vi "Parse Signal List.vi"(8 "error in (no error)":errorcluster, 11 "SwitchMatrix in":refnum<class "SwitchMatrix.lvclass">) -> (0 "error out":errorcluster, 3 "SwitchMatrix out":refnum<class "SwitchMatrix.lvclass">)   [LabVIEW 2019, in "SwitchMatrix.lvlib" / "SwitchMatrix.lvclass"]
uses:
  Library/SwitchMatrix.lvclass
  C:/Users/Public/Documents/Development/builds/Tools/Config.lvlibp/Config.lvclass
  Library/SwitchMatrix.lvclass/SwitchMatrix.ctl
  Accessors/Read Relay Name.vi
  builds/Tools/Config.lvlibp/Accessors/Read Device Signals.vi
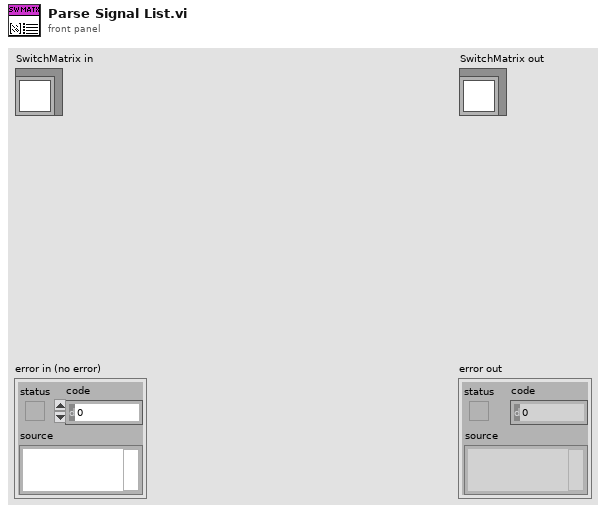
[diagram p1: front panel]
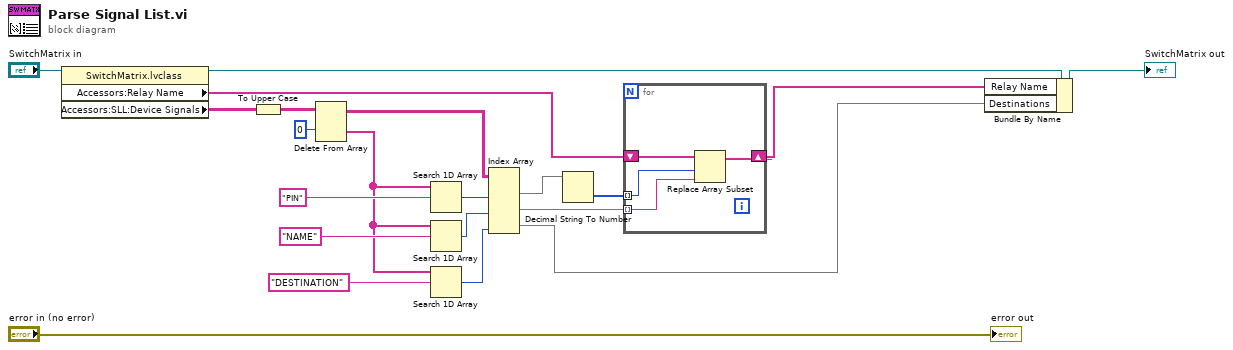
[diagram p0: block diagram]
diagram:
  n1 = property class="SwitchMatrix.lvclass"(reference="SwitchMatrix in") -> (reference out=w19:refnum<class "SwitchMatrix.lvclass">, "Accessors:Relay Name"=w12:string[], "Accessors:SLL:Device Signals"=w20:string[][])  [unwired: 1 in, 1 out]
  n2 = To Upper Case(1:w20) -> (0:w2:string[][])
  n3 = Delete From Array(array=w2, index (row)=0 ("disabled index (col)")) -> (deleted portion=w4:string[], array with subset deleted=w16:string[][])  [unwired: 2 in]
  n4 = Search 1D Array(1D array=w4, element="PIN") -> (index of element=w15:i32)  [unwired: 1 in]
  n5 = Search 1D Array(1D array=w4, element="NAME") -> (index of element=w14:i32)  [unwired: 1 in]
  n6 = Search 1D Array(1D array=w4, element="DESTINATION") -> (index of element=w5:i32)  [unwired: 1 in]
  n7 = Index Array(array=w16, index (col) #1=w15, index (col) #2=w14, index (col) #3=w5) -> (element #1=w11:string[], element #2=w9:string[], element #3=w1:string[])  [unwired: 3 in]
  n8 = Decimal String To Number(string=w11) -> (number=w10:i32[])  [unwired: 2 in, 1 out]
  n9 = for {
    tunnel: w10 -> [w22] mode=indexing
    tunnel: w9 -> [w23] mode=indexing
    shift-right: [w24] -> w6
    shift-left: w12 -> [w25]
    n10 = Replace Array Subset(array=w25, new element=w23, index=w22) -> (w24:string[])
  }
  n11 = Bundle By Name(cluster=w19, "Relay Name"=w6, "Destinations"=w1) -> (→"SwitchMatrix out":refnum<class "SwitchMatrix.lvclass">)
  "error out" <- "error in (no error)"
